vi "Generate Wave API.vi"(4 "RX.Data":u8[](array[numeric]), 6 "TX.Data":T1 caption="Transmission Data" format="%.0x", 8 "error in (no error)":errorcluster, 10 "Addr. Mode":refnum<data-value>, 11 "DVR IN":refnum<data-value>) -> (0 "error out":errorcluster, 3 "DVR OUT":refnum<data-value>)   [LabVIEW 2020, in "TX Speed.lvclass"]
uses:
  TX Speed.lvclass
  Addressing Mode/Parent/Addressing Mode.lvclass
  TypeDef/Transmission Data.ctl
  I2C Controller Lib.lvlib
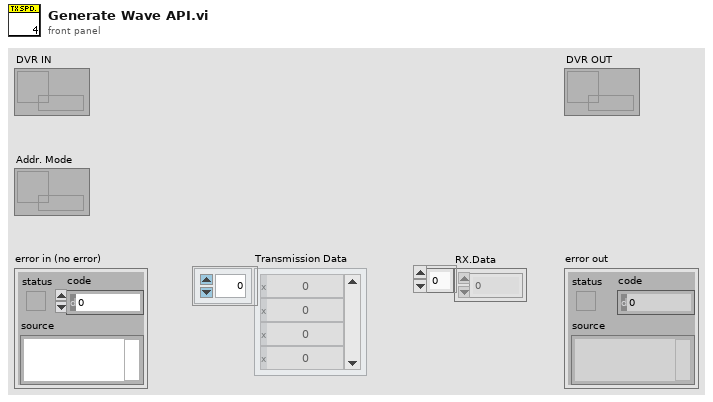
[diagram p1: front panel]
types:
  T1 = typedef "I2C Controller Lib.lvlib/Transmission Data.ctl" = u8[]
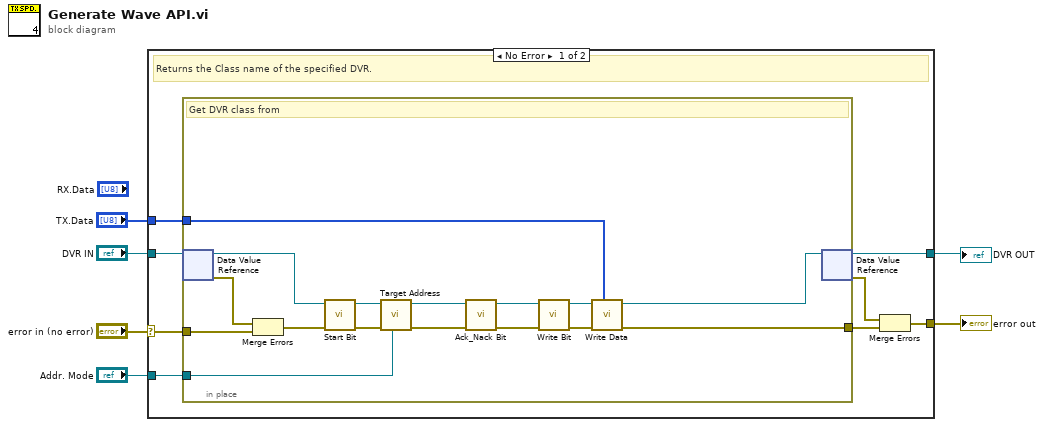
[diagram p0: block diagram]
diagram:
  n1 = case shown="No Error" "error in (no error)" {
    selector: "error in (no error)" -> [w13 w32]
    tunnel: [w14 w31] -> w3
    tunnel: [w11 w32] -> w5
    tunnel: "DVR IN" -> [w8 w31]
    tunnel: "Addr. Mode" -> [w10 _]
    tunnel: "TX.Data" -> [w7 _]
    frame No Error {
      # "Returns the Class name of the specified DVR."
      n2 = in-place {
        in-place-border: w13 -> [w30]
        in-place-border: w10 -> [w24]
        in-place-border: [w20] -> w9
        in-place-border: w7 -> [w19]
        # "Get DVR class from"
        n3 = in-place-dvr #1(w8) -> (w27:refnum<class "TX Speed.lvclass">, w29:errorcluster)
        n4 = Merge Errors(w29, w30) -> (w28:errorcluster)
        n5 = call-dynamic "Start Bit.vi"("error in (no error)"=w28, "TX Speed in"=w27) -> ("error out"=w25:errorcluster, "TX Speed out"=w26:refnum<class "TX Speed.lvclass">)  [unwired: 8 in]
        n6 = call-dynamic "Target Address.vi"("Addr. Mode"=w24, "error in (no error)"=w25, "TX Speed in"=w26) -> ("error out"=w17:errorcluster, "TX Speed out"=w18:refnum<class "TX Speed.lvclass">)  [unwired: 7 in]
        n7 = call-dynamic "Ack_Nack Bit.vi"("error in (no error)"=w17, "TX Speed in"=w18) -> ("error out"=w15:errorcluster, "TX Speed out"=w16:refnum<class "TX Speed.lvclass">)  [unwired: 8 in]
        n8 = call-dynamic "Write Bit.vi"("error in (no error)"=w15, "TX Speed in"=w16) -> ("error out"=w21:errorcluster, "TX Speed out"=w23:refnum<class "TX Speed.lvclass">)  [unwired: 8 in]
        n9 = call-dynamic "Write Data.vi"("TX.Data"=w19, "error in (no error)"=w21, "TX Speed in"=w23) -> ("error out"=w20:errorcluster, "TX Speed out"=w22:refnum<class "TX Speed.lvclass">)  [unwired: 7 in]
        n10 = in-place-dvr #1(w22) -> (w14:refnum<data-value>, w12:errorcluster)
      }
      n11 = Merge Errors(w12, w9) -> (w11:errorcluster)
    }
    frame Error {
    }
  }
  "error out" <- w5
  "DVR OUT" <- w3
